vi "Get MotionControl Devices List.vi"(8 "error in (no error)":errorcluster) -> (0 "error out":errorcluster, 2 "Device List":string[](array[string]), 3 "Device List Size":i16)   [LabVIEW 2017, in "XYStage.KIM101.lvclass"]
uses:
  XYStage.KIM101.lvclass
  D:/upwork/Laser Measurement Tool/Laser/project/data/Thorlabs.MotionControl.DeviceManagerCLI.dll
  data/Thorlabs.MotionControl.DeviceManagerCLI.dll
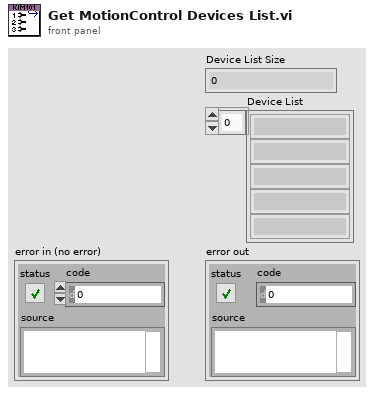
[diagram p1: front panel]
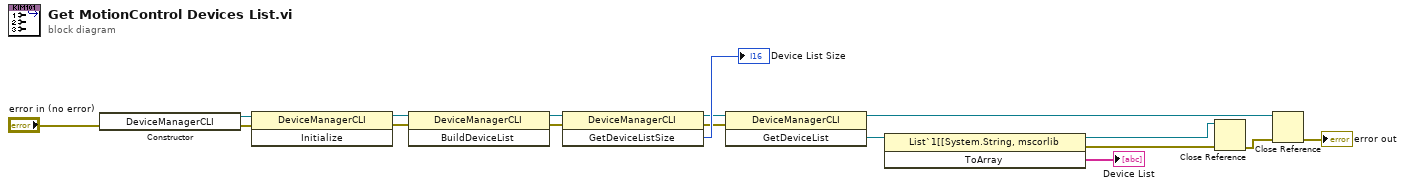
[diagram p0: block diagram]
diagram:
  n1 = constructor class="DeviceManagerCLI"(error in="error in (no error)") -> (reference out=w6:refnum<k24>, error out=w5:errorcluster)  [unwired: 2 in, 1 out]
  n2 = invoke class="DeviceManagerCLI" method="Initialize"(reference=w6, error in=w5) -> (reference out=w8:refnum<k24>, error out=w7:errorcluster)  [unwired: 1 in, 1 out]
  n3 = invoke class="DeviceManagerCLI" method="BuildDeviceList"(reference=w8, error in=w7) -> (reference out=w17:refnum<k24>, error out=w15:errorcluster)  [unwired: 1 in, 1 out]
  n4 = invoke class="DeviceManagerCLI" method="GetDeviceListSize"(reference=w17, error in=w15) -> (reference out=w14:refnum<k24>, error out=w13:errorcluster, "GetDeviceListSize"=→"Device List Size":i16)  [unwired: 1 in]
  n5 = invoke class="DeviceManagerCLI" method="GetDeviceList"(reference=w14, error in=w13) -> (reference out=w2:refnum<k24>, "GetDeviceList"=w12:refnum<k24>)  [unwired: 1 in, 1 out]
  n6 = invoke class="List`1[[System.String, mscorlib" method="ToArray"(reference=w12) -> (reference out=w10:refnum<k24>, error out=w9:errorcluster, "ToArray"=→"Device List":string[])  [unwired: 2 in]
  n7 = Close Reference(reference=w10, error in (no error)=w9) -> (error out=w3:errorcluster)
  n8 = Close Reference(reference=w2, error in (no error)=w3) -> (error out=→"error out":errorcluster)
